vi "Configure Waveform (Step).vi"(0 "VISA resource name":refnum<visa-resource-name>, 1 "Step Start Time (0.0 s)":dbl format="%^.3e", 2 "Step Start Level (0.0)":dbl format="%^.3e", 5 "Channel Name (1)":string="1", 9 "Waveform Type (1: Voltage)":i32(ring)=1 items=["Voltage"=1, "Current"=0], 11 "error in (no error)":errorcluster {"code" format="%.0x"}, 12 "Step End Time (0.0 s)":dbl format="%^.3e", 13 "Step End Level (0.0)":dbl format="%^.3e") -> (4 "VISA resource name out":refnum<visa-resource-name>, 15 "error out":errorcluster {"code" format="%.0x"})   [LabVIEW 2016, in "Agilent N6700 Series.lvlib"]
doc: "Configures the step waveform.\n\n<b>Note:</b>\nThis VI only applies to the N6705B and N6705C DC Power Analyzer."
uses:
  <instrlib>/Agilent N6700 Series/Agilent N6700 Series.lvlib
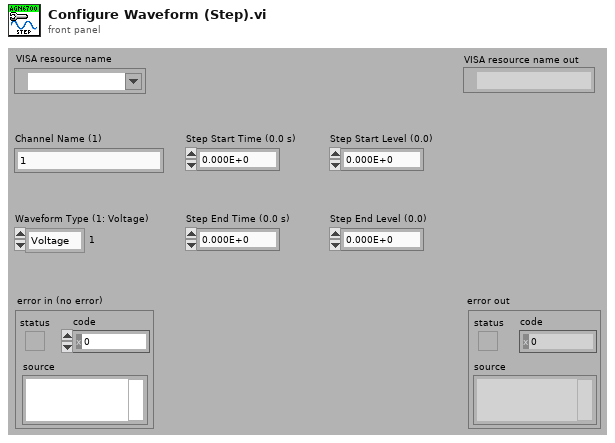
[diagram p1: front panel]
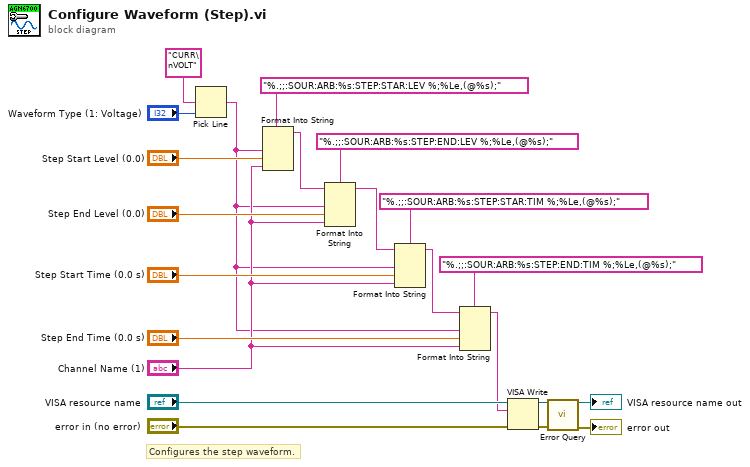
[diagram p0: block diagram]
diagram:
  # "Configures the step waveform."
  n1 = Pick Line(multi-line string="CURR\nVOLT", line index="Waveform Type (1: Voltage)") -> (output string=w1:string)  [unwired: 1 in]
  n2 = Format Into String(format string="%.;;:SOUR:ARB:%s:STEP:STAR:LEV %;%Le,(@%s);", w1, "Step Start Level (0.0)", "Channel Name (1)") -> (resulting string=w12:string)  [unwired: 2 in, 1 out]
  n3 = Format Into String(format string="%.;;:SOUR:ARB:%s:STEP:END:LEV %;%Le,(@%s);", initial string=w12, w1, "Step End Level (0.0)", "Channel Name (1)") -> (resulting string=w11:string)  [unwired: 1 in, 1 out]
  n4 = Format Into String(format string="%.;;:SOUR:ARB:%s:STEP:STAR:TIM %;%Le,(@%s);", initial string=w11, w1, "Step Start Time (0.0 s)", "Channel Name (1)") -> (resulting string=w4:string)  [unwired: 1 in, 1 out]
  n5 = Format Into String(format string="%.;;:SOUR:ARB:%s:STEP:END:TIM %;%Le,(@%s);", initial string=w4, w1, "Step End Time (0.0 s)", "Channel Name (1)") -> (resulting string=w3:string)  [unwired: 1 in, 1 out]
  n6 = VISA Write(VISA resource name="VISA resource name", write buffer=w3, error in (no error)="error in (no error)") -> (VISA resource name out=w18:refnum<visa-resource-name>, error out=w17:errorcluster)  [unwired: 1 out]
  n7 = call <instrlib>:"Error Query.vi"("VISA resource name"=w18, "error in (no error)"=w17) -> ("VISA resource name out"=→"VISA resource name out":refnum<visa-resource-name>, "error out"=→"error out":errorcluster)  [unwired: 10 in, 2 out]
